vi "IR Sensor.vi"(2 "Enum":enum16{"Start", "Run", "End"}(ring)) -> (0 "Voltage":dbl)   [LabVIEW 2014]
uses:
  TypeDefs/Analog Module 1.ctl
  <vilib>/Rock Robotics/SystemInterfaces/Typedef/FPGA_TypedefAnalogModule.ctl
  <vilib>/Rock Robotics/SystemInterfaces/AI/FPGA_AIChannel.ctl
panel:
  in  "Analog Module A":T1={"Module"=enum."Analog Module 1", "Gyro"=enum."AI 1", "IR Sensor"=enum."AI 2", "Unassigned"=enum."AI 3", "Unassigned"=enum."AI 3", "Unassigned"=enum."AI 5", "Unassigned"=enum."AI 6", "Unassigned"=enum."AI 7", "Unassigned"=enum."AI 8"}
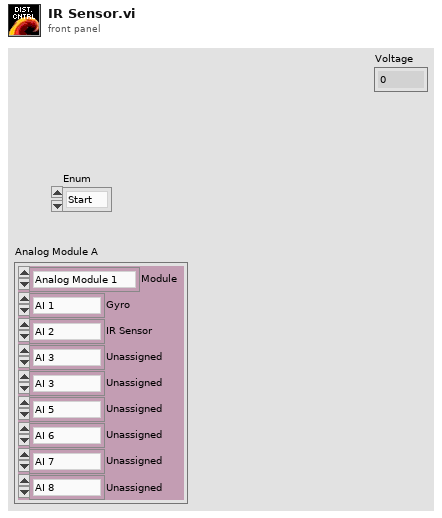
[diagram p1: front panel]
types:
  T1 = typedef "Analog Module 1.ctl" = cluster{"Module":T2, "Gyro":T3, "IR Sensor":T3, "Unassigned":T3, "Unassigned":T3, "Unassigned":T3, "Unassigned":T3, "Unassigned":T3, "Unassigned":T3}
  T2 = typedef "FPGA_TypedefAnalogModule.ctl" = enum16{"Analog Module 1", "Analog Module 2"}
  T3 = typedef "FPGA_AIChannel.ctl" = enum8{"AI 1", "AI 2", "AI 3", "AI 4", "AI 5", "AI 6", "AI 7", "AI 8", "Invalid"}
  T4 = typedef "WPI_AnalogChannelDevRef.ctl" = cluster{"DevStatus":errorcluster, "Analog Module":T2, "Analog Channel":T3}
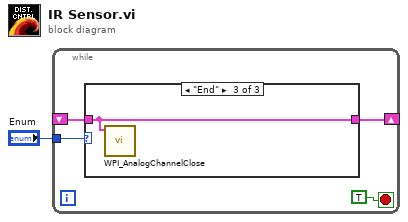
[diagram p0: block diagram]
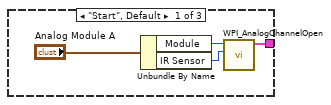
[diagram p2: hidden frame]
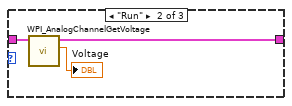
[diagram p3: hidden frame]
diagram:
  n1 = while {
    tunnel: "Enum" -> [w4]
    shift-right: [w2] -> _
    shift-left: _ -> [w3]
    stop <- TRUE stop-if-true
    n2 = case shown="\"End\"" w4 {
      tunnel: w3 -> [_ w12 w13]
      tunnel: [w6 w11 w13] -> w2
      frame "Start", Default {
        n3 = Unbundle By Name("Analog Module A") -> ("Module"=w8:T2, "IR Sensor"=w7:T3)
        n4 = call <vilib>:"WPI_AnalogChannelOpen.vi"("Analog Channel"=w7, "Analog Module (Module 1)"=w8) -> ("AIDeviceRef"=w6:T4)  [unwired: 8 in, 1 out]
      }
      frame "Run" {
        n5 = call <vilib>:"WPI_AnalogChannelGetVoltage.vi"("AIDeviceRef"=w12) -> ("Voltage"=→"Voltage":dbl, "AIDeviceRef"=w11:T4)  [unwired: 8 in, 1 out]
      }
      frame "End" {
        n6 = call <vilib>:"WPI_AnalogChannelClose.vi"("AIDeviceRef"=w13) -> ()  [unwired: 10 in, 1 out]
      }
    }
  }
